vi "TL_read_next_task.vi"(3 "error in":errorcluster, 5 "Time lapse parameters":T2) -> (0 "error out":errorcluster, 1 "task":T1, 2 "Time lapse parameters":T2)   [LabVIEW 2015]
uses:
  CONTROLS/Q_main_element.ctl
  GLOBAL/Global_ABORT.vi
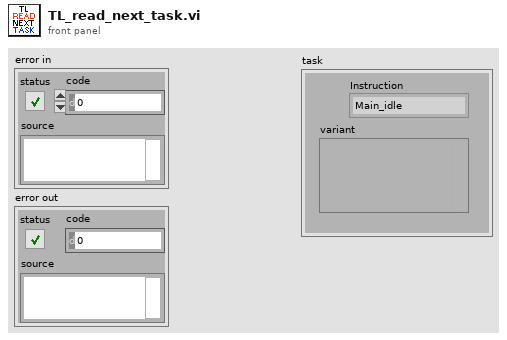
[diagram p1: front panel]
types:
  T1 = typedef "Q_main_element.ctl" = cluster{"variant":variant, "Instruction":enum16{"Main_idle", "Main_initialize", "Main_initialize_TDMS", "Main_initialize_Queue", "Main_error", "Main_DAQ_initialization_results", "Main_ASI_initialization_results", "Main_Piezo_initialization_results", "Main_Valve_initialization_results", "Main_Pump_initialization_results", "Main_CAMERA_initialization_results", "Main_DAQ_error", "Main_ASI_error", "Main_Piezo_error", "Main_CAMERA_error", "Main_Valve_error", "Main_Pump_error", "Main_start_acquiring", "Main_not_acquiring", "Main_acquiring", "Main_stop_acquiring", "Main_change_exposure", "Main_change_z_scan_parameters", "Main_define_ROI", "Main_read_kinetic_time", "Main_cooler", "Main_read_temperature", "Main_save_XY", "Main_load_XY", "Main_discard_XY", "Main_move_to_XY", "Main_measure_QPD", "Main_autofocus_calibration", "Main_save_PID", "Main_change_H_valve_position", "Main_two_way_valve", "Main_save_movie", "Main_init_single_scan", "Main_single_scan", "Main_stop_single_scan", "Main_merFISH_illumination_parameters", "Main_merFISH_buffer_probe_list", "Main_merFISH_injections_procedure", "Main_merFISH_save_setpoint", "Main_merFISH_init", "Main_merFISH_resume", "Main_merFISH_start_autofocus", "Main_merFISH_open_close_valve_merFISH", "Main_merFISH_open_close_valve_photobleaching", "Main_merFISH_hybridization", "Main_merFISH_move_to_ROI", "Main_merFISH_wait_stabilization", "Main_merFISH_scan", "Main_merFISH_photobleaching_injection", "Main_merFISH_photobleaching", "Main_merFISH_save", "Main_merFISH_send_email", "Main_merFISH_close", "Main_TL_define_parameters", "Main_TL_init", "Main_TL_start_autofocus", "Main_TL_move_to_ROI", "Main_TL_wait_for_stabilization", "Main_TL_scan", "Main_TL_wait_cycle_end", "Main_TL_close", "Main_STOP"}}
  T2 = cluster{"TL - setpoint cluster":cluster{"405":dbl[], "488":dbl[], "561":dbl[], "640":dbl[], "BF":dbl[]}, "# repetitions":i32, "TL array":dbl[][], "ROIs":dbl[][], "TL movie path":path, "# cycle":i32, "t0":dbl, "t0 experiment":dbl, "Task list template":T1[], "Task list":T1[], "slope":dbl}
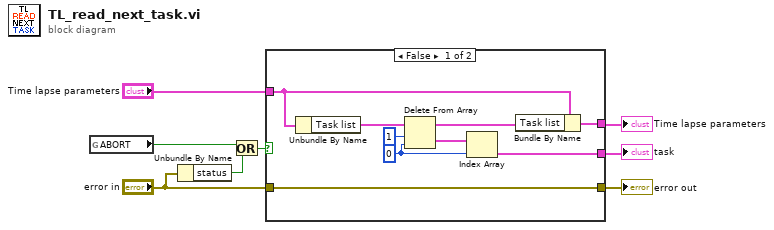
[diagram p0: block diagram]
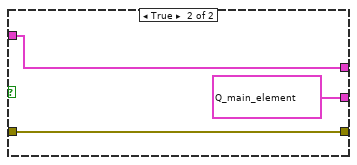
[diagram p2: hidden frame]
diagram:
  n1 = global read "Global_ABORT.vi" "ABORT"() -> (w3:bool)
  n2 = Unbundle By Name("error in") -> ("status"=w4:bool)
  n3 = Or(x=w3, y=w4) -> (x .or. y?=w5:bool)
  n4 = case shown="False" w5 {
    tunnel: [w13 T1 {"variant"=variant, "Instruction"=enum."Main_TL_close"} ("element")] -> w8
    tunnel: "Time lapse parameters" -> [w12 w19]
    tunnel: [w11 w19] -> w2
    tunnel: "error in" -> [w10 w20]
    tunnel: [w10 w20] -> w7
    frame False {
      w17 = 0 ("index")
      n5 = Unbundle By Name(w12) -> ("Task list"=w14:T1[])
      n6 = Delete From Array(array=w14, length=1, index=w17) -> (deleted portion=w16:T1[], array with subset deleted=w9:T1[])
      n7 = Index Array(array=w16, index=w17) -> (element=w13:T1)
      n8 = Bundle By Name(cluster=w12, "Task list"=w9) -> (w11:T2)
    }
    frame True {
    }
  }
  "task" <- w8
  "error out" <- w7
  "Time lapse parameters" <- w2
